vi "List of uServices to launch at startup.vi"(8 "error in (no error)":errorcluster, 11 "Guardian in":refnum<class "Guardian.lvclass">) -> (0 "error out":errorcluster, 2 "Array":string[](array[string]), 3 "Guardian out":refnum<class "Guardian.lvclass">)   [LabVIEW 2026, in "TALOS.lvlib" / "Guardian.lvlib" / "Guardian.lvclass"]
uses:
  Guardian.lvclass
  C:/LabVIEW Code/TALOS/talos/Ancestor/Ancestor/Ancestor.lvclass
  Ancestor/Ancestor/Ancestor.lvclass/Ancestor.ctl
  Ancestor/Ancestor/Read ID.vi
  Support VIs/Global Constants.vi
  Support VIs/Global Memory.vi
  TALOS.lvlib
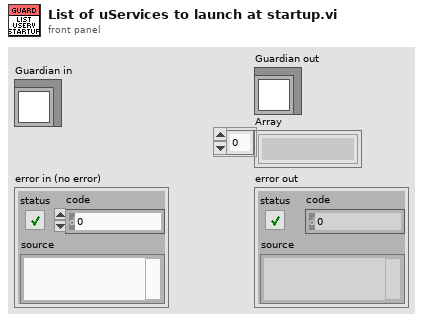
[diagram p1: front panel]
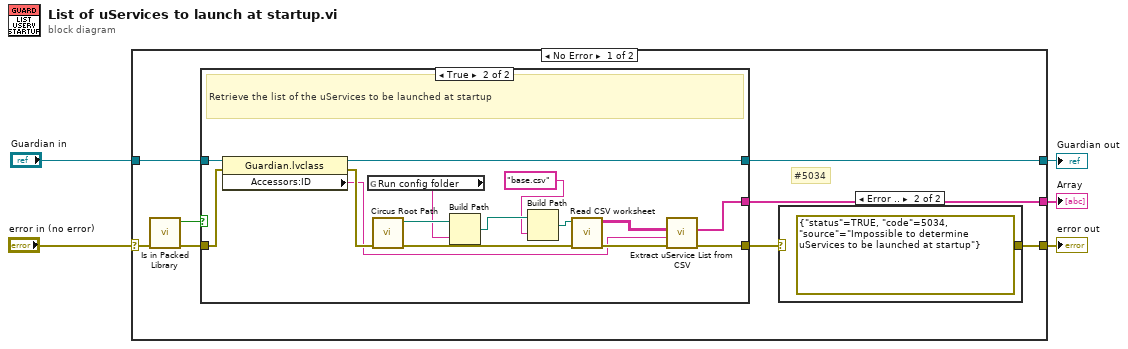
[diagram p0: block diagram]
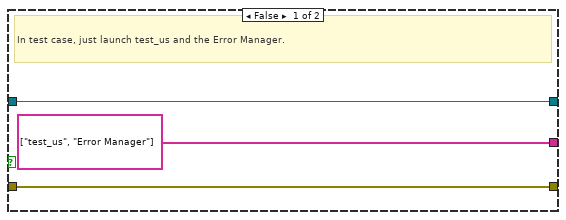
[diagram p2: hidden frame]
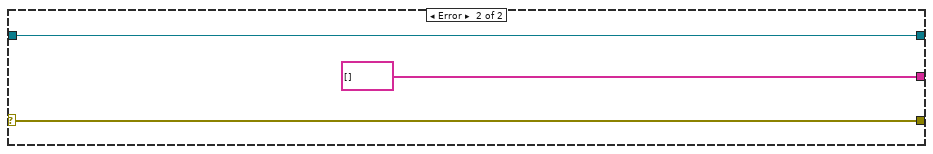
[diagram p4: hidden frame]
diagram:
  n1 = case shown="No Error" "error in (no error)" {
    selector: "error in (no error)" -> [w12 w36]
    tunnel: [w13 string[] []] -> w5
    tunnel: [w8 w36] -> w4
    tunnel: "Guardian in" -> [w9 w34]
    tunnel: [w6 w34] -> w1
    frame No Error {
      # "#5034"
      n2 = call "Is in Packed Library.vi"("error in (no error)"=w12) -> ("error out"=w11:errorcluster, "Is In Packed Library"=w10:bool)  [unwired: 9 in]
      n3 = case shown="True" w10 {
        tunnel: [string[] ["test_us", "Error Manager"] w22] -> w13
        tunnel: w11 -> [w15 w19]
        tunnel: [w15 w25] -> w7
        tunnel: w9 -> [w14 w21]
        tunnel: [w14 w20] -> w6
        frame False {
          # "In test case, just launch test_us and the Error Manager."
        }
        frame True {
          # "Retrieve the list of the uServices to be launched at startup"
          n4 = property class="Guardian.lvclass"(reference=w21, error in=w19) -> (reference out=w20:refnum<class "Guardian.lvclass">, error out=w18:errorcluster, "Accessors:ID"=w17:string)
          n5 = global read "Global Constants.vi" "Run config folder"() -> (w24:string)
          n6 = call "Circus Root Path.vi"("error in (no error)"=w18) -> ("error out"=w28:errorcluster, "Circus Root Path"=w27:path)  [unwired: 9 in]
          n7 = Build Path(base path=w27, name or relative path=w24) -> (appended path=w29:path)
          n8 = Build Path(base path=w29, name or relative path="base.csv") -> (appended path=w30:path)
          n9 = call "Read CSV worksheet.vi"("error in (no error)"=w28, "appended path"=w30) -> ("error out"=w31:errorcluster, "Sheet"=w23:string[][])  [unwired: 8 in]
          n10 = call "Extract uService List from CSV.vi"("error in (no error)"=w31, "Guardian ID"=w17, "CSV table"=w23) -> ("error out"=w25:errorcluster, "uS array"=w22:string[])  [unwired: 7 in]
        }
      }
      n11 = case shown="Error .." w7 {
        selector: w7 -> [w32 _]
        tunnel: [w32 errorcluster {"status"=TRUE, "code"=5034, "source"="Impossible to determine uServices to be launched at startup"} ("error IO")] -> w8
        frame No Error {
        }
        frame Error {
        }
      }
    }
    frame Error {
    }
  }
  "Array" <- w5
  "error out" <- w4
  "Guardian out" <- w1
